vi "9265 4Ch Analog Output.vi"(2 "Packets":u64[](array[numeric])=[0, 0], 4 "9265 I/O":T1={"AO0"="Chassis1/Mod2/AO0", "AO1"="Chassis1/Mod2/AO1", "AO2"="Chassis1/Mod2/AO1", "AO3"="Chassis1/Mod2/AO0"}) -> ()   [LabVIEW 2010]
uses:
  <vilib>/eio/EIONode/EIONode.xnode
  <vilib>/rvi/eio/nirviEIOImplementation/nirviEIOImplementation.xnode
  <vilib>/rvi/eio/common/nirviEmuClasses.ctl
  <vilib>/rvi/eio/common/nirviEmuTemplateMethod_noerrors.vi
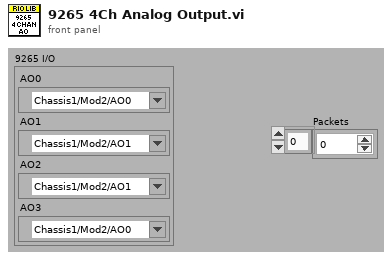
[diagram p1: front panel]
types:
  T1 = cluster{"AO0":refnum<k21>, "AO1":refnum<k21>, "AO2":refnum<k21>, "AO3":refnum<k21>}
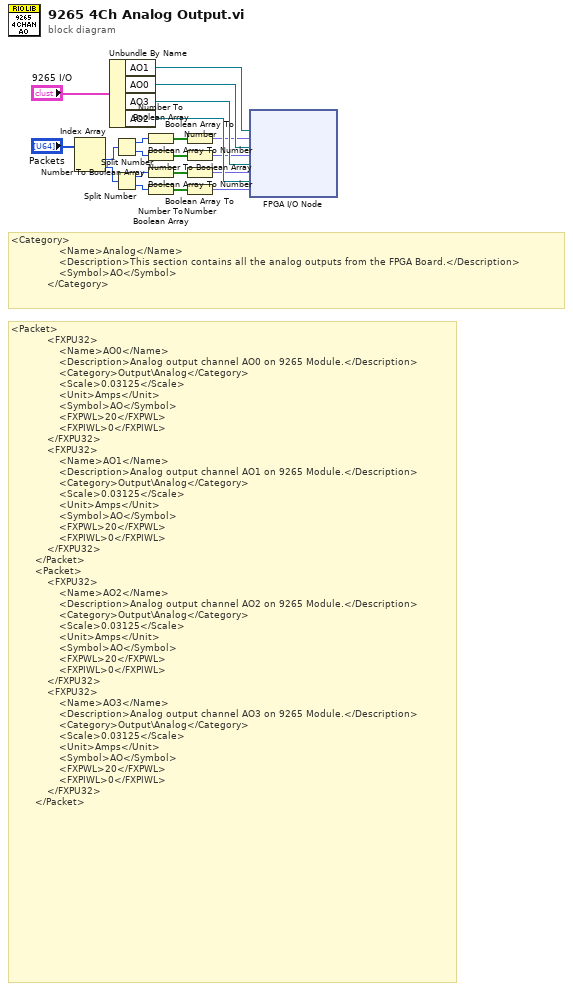
[diagram p0: block diagram]
diagram:
  # "<Category>\n                <Name>Analog</Name>\n                <Description>This section contains all the analog outputs from the FPGA Board.</Description>\n                <Symbol>AO</Symbol>\n            </Category>"
  # "<Packet>\n            <FXPU32>\n                <Name>AO0</Name>\n                <Description>Analog output channel AO0 on 9265 Module.</Description>\n                <Category>Output\\Analog</Category>\n                <Scale>0.03125</Scale>\n                <Unit>Amps</Unit>\n                <Symbol>AO</Symbol>\n                <FXPWL>20</FXPWL>\n                <FXPIWL>0</FXPIWL>\n            </FXPU32>\n            <FXPU32>\n                <Name>AO1</Name>\n                <Description>Analog output channel AO1 on 9265 Module.</Description>\n                <Category>Output\\Analog</Category>\n                <Scale>0.03125</Scale>\n                <Unit>Amps</Unit>\n                <Symbol>AO</Symbol>\n                <FXPWL>20</FXPWL>\n                <FXPIWL>0</FXPIWL>\n            </FXPU32>\n        </Packet>\n        <Packet>\n            <FXPU32>\n                <Name>AO2</Name>\n                <Description>Analog output channel AO2 on 9265 Module.</Description>\n                <Category>Output\\Analog</Category>\n                <Scale>0.03125</Scale>\n                <Unit>Amps</Unit>\n                <Symbol>AO</Symbol>\n                <FXPWL>20</FXPWL>\n                <FXPIWL>0</FXPIWL>\n            </FXPU32>\n            <FXPU32>\n                <Name>AO3</Name>\n                <Description>Analog output channel AO3 on 9265 Module.</Description>\n                <Category>Output\\Analog</Category>\n                <Scale>0.03125</Scale>\n                <Unit>Amps</Unit>\n                <Symbol>AO</Symbol>\n                <FXPWL>20</FXPWL>\n                <FXPIWL>0</FXPIWL>\n            </FXPU32>\n        </Packet>"
  n1 = Index Array(array="Packets") -> (element #1=w8:u64, element #2=w9:u64)  [unwired: 2 in]
  n2 = Unbundle By Name("9265 I/O") -> ("AO1"=w19:refnum<k21>, "AO0"=w20:refnum<k21>, "AO3"=w18:refnum<k21>, "AO2"=w17:refnum<k21>)
  n3 = Split Number(x=w8) -> (hi(x)=w10:u32, lo(x)=w11:u32)
  n4 = Split Number(x=w9) -> (hi(x)=w12:u32, lo(x)=w13:u32)
  n5 = Number To Boolean Array(number=w10) -> (Boolean array=w15:bool[])
  n6 = Number To Boolean Array(number=w11) -> (Boolean array=w6:bool[])
  n7 = Number To Boolean Array(number=w12) -> (Boolean array=w4:bool[])
  n8 = Number To Boolean Array(number=w13) -> (Boolean array=w3:bool[])
  n9 = Boolean Array To Number(Boolean array=w15) -> (number=w14:fxp<+,20,-5>)
  n10 = Boolean Array To Number(Boolean array=w6) -> (number=w5:fxp<+,20,-5>)
  n11 = Boolean Array To Number(Boolean array=w4) -> (number=w1:fxp<+,20,-5>)
  n12 = Boolean Array To Number(Boolean array=w3) -> (number=w2:fxp<+,20,-5>)
  n13 = xnode "FPGA I/O Node"("I/O Item"=w14, "I/O Item"=w5, "I/O Item"=w1, "I/O Item"=w2, "FPGA I/O In"=w19, "FPGA I/O In"=w20, "FPGA I/O In"=w18, "FPGA I/O In"=w17) -> ()  [unwired: 4 out]
